vi "PQconnectdb.vi"(8 "error in (no error)":errorcluster, 11 "conninfo":string) -> (0 "error out":errorcluster, 3 "conn":u32)   [LabVIEW 2018, in "libpqlv.lvlib"]
doc: "Makes a new connection to the database server."
uses:
  libpqlv.lvlib
  lib/libpq.dll
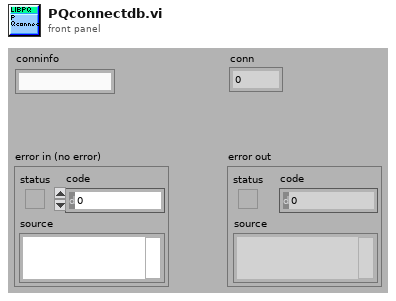
[diagram p1: front panel]
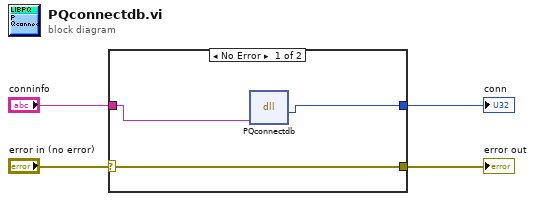
[diagram p0: block diagram]
diagram:
  n1 = case shown="No Error" "error in (no error)" {
    selector: "error in (no error)" -> [w7 w8]
    tunnel: [w7 w8] -> w3
    tunnel: [w6 _] -> w2
    tunnel: "conninfo" -> [w5 _]
    frame No Error {
      n2 = dll-call lib="D:/Users/erics/Documents/TC-3/DAQ/PostgreSQL2LabVIEW/libpqlv/lib/libpq.*" fn="PQconnectdb"("conninfo"=w5) -> ("conn"=w6:u32)  [unwired: 4 in, 2 out]
    }
    frame Error {
    }
  }
  "conn" <- w2
  "error out" <- w3
